vi "Waveform_Find Time Range.vi"(7 "Open Interval? (T)":bool, 9 "Waveform 2":T1, 11 "Waveform 1":T1) -> (2 "Max Tf Out":timestamp, 3 "Min T0 Out":timestamp)   [LabVIEW 2020]
uses:
  Universal Controls/Waveform_Data.ctl
  <vilib>/Waveform/WDTOps.llb/WDT Get Final Time Value DBL.vi
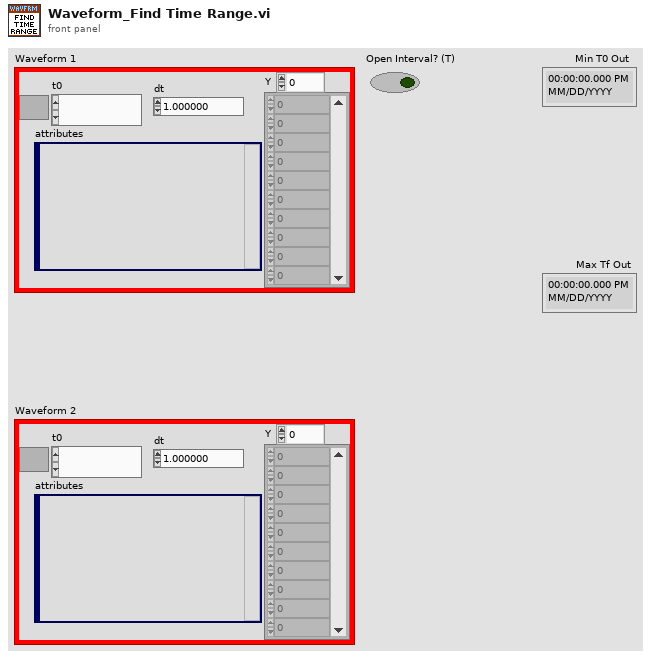
[diagram p1: front panel]
types:
  T1 = typedef "Waveform_Data.ctl" = waveform(dbl)
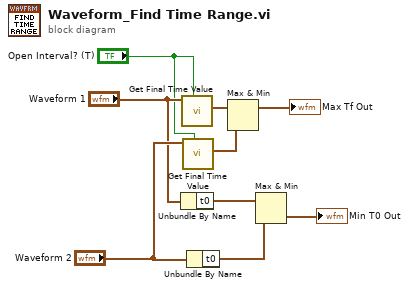
[diagram p0: block diagram]
diagram:
  n1 = Unbundle By Name("Waveform 1") -> ("t0"=w7:timestamp)
  n2 = call-poly <vilib>:"Get Final Time Value.vi"("open interval? (T)"="Open Interval? (T)", "waveform in"="Waveform 1") -> ("tf"=w4:timestamp)  [unwired: 7 in, 2 out]
  n3 = call-poly <vilib>:"Get Final Time Value.vi"("open interval? (T)"="Open Interval? (T)", "waveform in"="Waveform 2") -> ("tf"=w5:timestamp)  [unwired: 7 in, 2 out]
  n4 = Unbundle By Name("Waveform 2") -> ("t0"=w9:timestamp)
  n5 = Max & Min(x=w4, y=w5) -> (max(x,y)=→"Max Tf Out":timestamp)  [unwired: 1 out]
  n6 = Max & Min(x=w7, y=w9) -> (min(x,y)=→"Min T0 Out":timestamp)  [unwired: 1 out]
